vi "Test Pass if Numeric Argument Incorrect and then Correct.vi"(8 "error in (no error)":errorcluster, 11 "Test Case In":refnum<class "Responsive Mock One Expectation Test.lvclass">) -> (0 "error out":errorcluster, 3 "Test Case Out":refnum<class "Responsive Mock One Expectation Test.lvclass">)   [LabVIEW 2020, in "Responsive Mock One Expectation Test.lvclass"]
uses:
  Responsive Mock One Expectation Test.lvclass
  C:/Program Files (x86)/National Instruments/LabVIEW 2020/vi.lib/Astemes/LUnit/Test Case.lvclass
  Test Doubles/Test Interface Responsive Mock/Test Interface Mock.lvclass
  C:/git/astemes-lmock/source/Framework/Mock/Mock.lvclass
  source/Expectations/One/One Identical Inputs.vi
  Responsive Mock One Expectation Test.lvclass/Responsive Mock One Expectation Test.ctl
  source/Expectations/One/One.lvclass
  Expectation Test/Responsive Mock Expectation Test.lvclass
  C:/git/astemes-lmock/tests/Expectation Test/Responsive Mock Expectation Test.lvclass
  C:/Program Files (x86)/National Instruments/LabVIEW 2020/vi.lib/Astemes/LUnit/LUnit Runnable.lvclass
  C:/git/astemes-lmock/tests/One Expectation Test/Responsive Mock One Expectation Test.lvclass
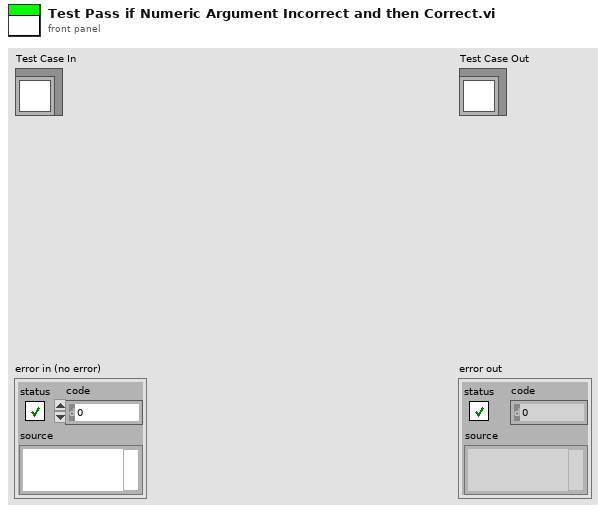
[diagram p1: front panel]
types:
  T1 = enum16{"", "Passed", "Failed", "Error", "Skipped", "Setup Error", "Broken", "Teardown Error"}
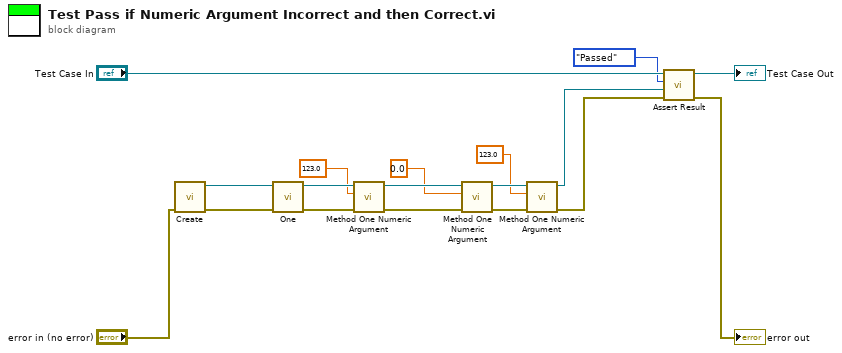
[diagram p0: block diagram]
diagram:
  n1 = call "Create.vi"("error in (no error)"="error in (no error)") -> ("error out"=w17:errorcluster, "Test Interface Mock Out"=w18:refnum<class "Test Interface Mock.lvclass">)  [unwired: 9 in]
  n2 = call-poly "One.vi"("error in (no error)"=w17, "Mock in"=w18) -> ("error out"=w15:errorcluster, "Mock out"=w16:refnum<class "Test Interface Mock.lvclass">)  [unwired: 8 in]
  n3 = call-dynamic "Method One Numeric Argument.vi"("error in (no error)"=w15, "Numeric"=123.0, "Test Interface Mock In"=w16) -> ("error out"=w14:errorcluster, "Test Interface Mock Out"=w8:refnum<class "Test Interface Mock.lvclass">)  [unwired: 7 in]
  n4 = call-dynamic "Method One Numeric Argument.vi"("error in (no error)"=w14, "Numeric"=0.0, "Test Interface Mock In"=w8) -> ("error out"=w9:errorcluster, "Test Interface Mock Out"=w6:refnum<class "Test Interface Mock.lvclass">)  [unwired: 7 in]
  n5 = call-dynamic "Method One Numeric Argument.vi"("error in (no error)"=w9, "Numeric"=123.0, "Test Interface Mock In"=w6) -> ("error out"=w3:errorcluster, "Test Interface Mock Out"=w2:refnum<class "Test Interface Mock.lvclass">)  [unwired: 7 in]
  n6 = call "Assert Result.vi"("error in (no error)"=w3, "Mock"=w2, "Status"=T1."Passed", "LUnit Test Case In"="Test Case In") -> ("error out"=→"error out":errorcluster, "LUnit Test Case Out"=→"Test Case Out":refnum<class "Responsive Mock One Expectation Test.lvclass">)  [unwired: 6 in]
